vi "DataSender.vi"(0 "Data":string, 1 "Action":string, 2 "ID":u32) -> ()   [LabVIEW 2025]
uses:
  ServerNetworkInterfaceGlobalVariables.vi
  ServerGlobalVariables.vi
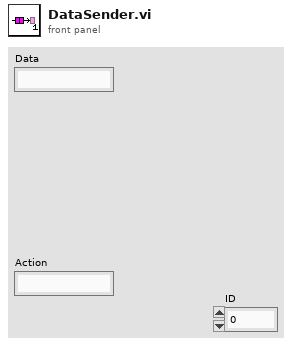
[diagram p1: front panel]
types:
  T1 = cluster{"Action":string, "seconds since 1Jan1904":timestamp, "Data":string}
  T2 = cluster{"Data":string, "Address":u32, "Port":u16}
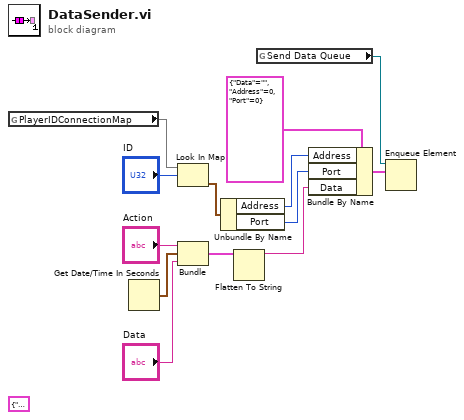
[diagram p0: block diagram]
diagram:
  (unwired) T1 {"Action"="", "seconds since 1Jan1904"=timestamp(0 s since 1904-01-01), "Data"=""} ("output cluster")
  n1 = global read "ServerGlobalVariables.vi" "PlayerIDConnectionMap"() -> (w4:map{u32, cluster{"Address":u32, "Port":u16}})
  n2 = Get Date/Time In Seconds() -> (seconds since 1Jan1904=w1:timestamp)
  n3 = Look In Map(map=w4, key="ID") -> (value=w2:cluster{"Address":u32, "Port":u16})  [unwired: 1 in, 1 out]
  n4 = Bundle("Action"="Action", "seconds since 1Jan1904"=w1, "Data"="Data") -> (w12:T1)  [unwired: 1 in]
  n5 = Unbundle By Name(w2) -> ("Address"=w5:u32, "Port"=w6:u16)
  n6 = Flatten To String(anything=w12) -> (data string=w13:string)  [unwired: 3 in, 2 out]
  n7 = global read "ServerNetworkInterfaceGlobalVariables.vi" "Send Data Queue"() -> (w7:refnum<queue>)
  n8 = Bundle By Name(cluster=T2 {"Data"="", "Address"=0, "Port"=0}, "Address"=w5, "Port"=w6, "Data"=w13) -> (w9:T2)
  n9 = Enqueue Element(queue=w7, element=w9) -> ()  [unwired: 2 in, 3 out]
